vi "PH_Cam_BaseClass.publish Image.vi"(1 "Notifier":refnum<notifier>, 2 "Image In":T1, 5 "error in (no error)":errorcluster) -> (16 "Image Out":T1, 19 "error out":errorcluster)   [LabVIEW 2014, in "PH_Cam_BaseClass.lvlib"]
doc: "This VI published the new image location by sending a notifier."
uses:
  <vilib>/vision/Image Controls.llb/IMAQ Image.ctl
  PH_Cam_BaseClass.lvlib
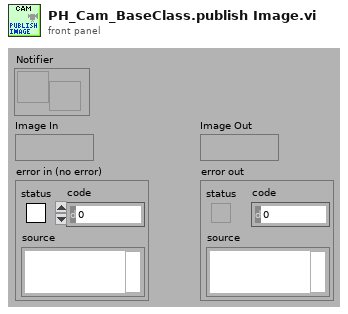
[diagram p1: front panel]
types:
  T1 = typedef "IMAQ Image.ctl" = refnum<image>
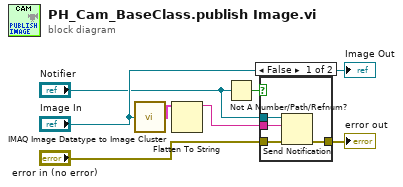
[diagram p0: block diagram]
diagram:
  n1 = call <vilib>:"IMAQ Image Datatype to Image Cluster.vi"("Image"="Image In") -> ("Image (dup)"=w3:cluster{string, u32})
  n2 = Flatten To String(anything=w3) -> (data string=w4:string)  [unwired: 3 in, 2 out]
  n3 = Not A Number/Path/Refnum?(number/path/refnum="Notifier") -> (NaN/Path/Refnum?=w1:bool)
  n4 = case shown="False" w1 {
    tunnel: [w11 w12] -> w7
    tunnel: "error in (no error)" -> [w10 w12]
    tunnel: w4 -> [w9 _]
    tunnel: "Notifier" -> [w8 _]
    frame False {
      n5 = Send Notification(notification=w9, notifier=w8, error in (no error)=w10) -> (error out=w11:errorcluster)  [unwired: 1 out]
    }
    frame True {
    }
  }
  "error out" <- w7
  "Image Out" <- "Image In"
